vi "To String.vi"(8 "error in (no error)":errorcluster, 11 "NT Scalar in":refnum<class "NT Scalar.lvclass">) -> (0 "error out":errorcluster, 2 "string":string, 3 "NT Scalar out":refnum<class "NT Scalar.lvclass">)   [LabVIEW 2020, in "PV Access.lvlib" / "PV Data.lvlib" / "NT Scalar.lvclass"]
uses:
  NT Scalar.lvclass
  NT Scalar.lvclass/NT Scalar.ctl
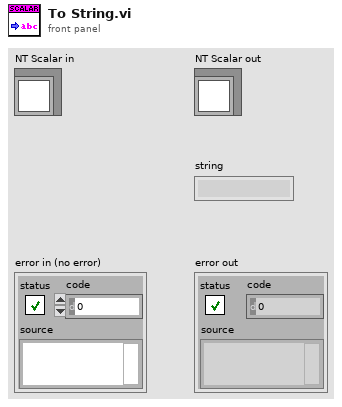
[diagram p1: front panel]
types:
  T1 = typedef "PV Access.lvlib/PV Data.lvlib/Type Code.ctl" = enum8{"Null", "Bool", "BoolA", "Int8", "Int8A", "Int16", "Int16A", "Int32", "Int32A", "Int64", "Int64A", "UInt8", "UInt8A", "UInt16", "UInt16A", "UInt32", "UInt32A", "UInt64", "UInt64A", "Float32", "Float32A", "Float64", "Float64A", "String", "StringA", "Struct", "StructA", "Union", "UnionA", "Any", "AnyA"}
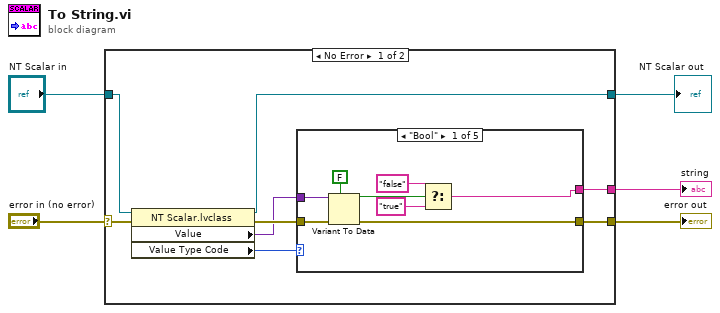
[diagram p0: block diagram]
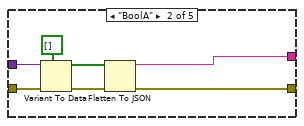
[diagram p2: hidden frame]
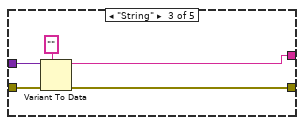
[diagram p3: hidden frame]
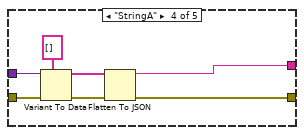
[diagram p4: hidden frame]
diagram:
  n1 = case shown="No Error" "error in (no error)" {
    selector: "error in (no error)" -> [w7 w43]
    tunnel: [w6 w43] -> w1
    tunnel: [w11 w42] -> w3
    tunnel: "NT Scalar in" -> [w13 w42]
    tunnel: [w8 _] -> w2
    frame No Error {
      n2 = property class="NT Scalar.lvclass"(reference=w13, error in=w7) -> (reference out=w11:refnum<class "NT Scalar.lvclass">, error out=w12:errorcluster, "Value"=w9:variant, "Value Type Code"=w10:T1)
      n3 = case shown="\"Bool\"" w10 {
        tunnel: w12 -> [w20 w27 w32 w39 w41]
        tunnel: w9 -> [w21 w28 w33 w40 _]
        tunnel: [w19 w23 w31 w35 w41] -> w6
        tunnel: [w14 w22 w29 w34 _] -> w8
        frame "Bool" {
          n4 = Variant To Data(error in=w20, type=FALSE, Variant=w21) -> (data=w17:bool, error out=w19:errorcluster)
          n5 = Select(t="false", s=w17, f="true") -> (s? t:f=w14:string)
        }
        frame "BoolA" {
          n6 = Variant To Data(error in=w27, type=bool[] [], Variant=w28) -> (data=w24:bool[], error out=w25:errorcluster)
          n7 = Flatten To JSON(anything=w24, error in (no error)=w25) -> (JSON string=w22:string, 11:w23:errorcluster)  [unwired: 1 in]
        }
        frame "String" {
          n8 = Variant To Data(error in=w32, type="", Variant=w33) -> (data=w29:string, error out=w31:errorcluster)
        }
        frame "StringA" {
          n9 = Variant To Data(error in=w39, type=string[] [], Variant=w40) -> (data=w36:string[], error out=w37:errorcluster)
          n10 = Flatten To JSON(anything=w36, error in (no error)=w37) -> (JSON string=w34:string, 11:w35:errorcluster)  [unwired: 1 in]
        }
        frame Default {
        }
      }
    }
    frame Error {
    }
  }
  "error out" <- w1
  "NT Scalar out" <- w3
  "string" <- w2
